vi "replaceTokens.vi"(8 "error in (no error)":errorcluster, 10 "Querry In":string, 11 "Goal in":refnum<class "Goal.lvclass">) -> (0 "error out":errorcluster, 2 "Query Out":string, 3 "Goal out":refnum<class "Goal.lvclass">)   [LabVIEW 2018, in "Goal.lvclass"]
uses:
  Goal.lvclass
  C:/GitRepos/Filthy-Lucre-Budgetizer/source/support/classes/UserEditableAmount/UserEditableAmount.lvclass
  Goal.lvclass/Goal.ctl
  WhichMonth/WhichMonth.lvclass
  Category/Category.lvclass
  UserEditableAmount/UserEditableAmount.lvclass
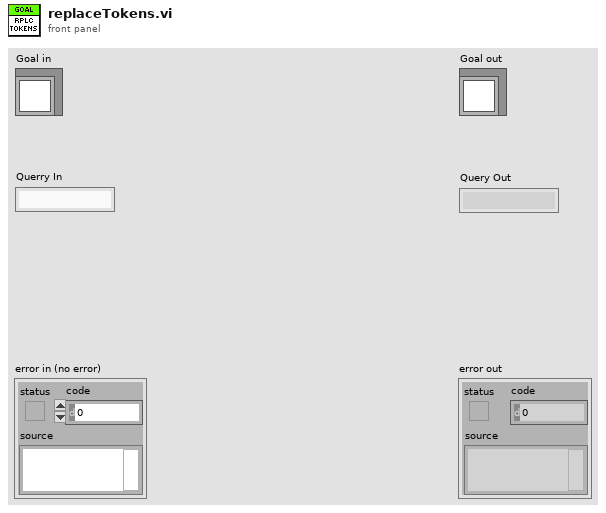
[diagram p1: front panel]
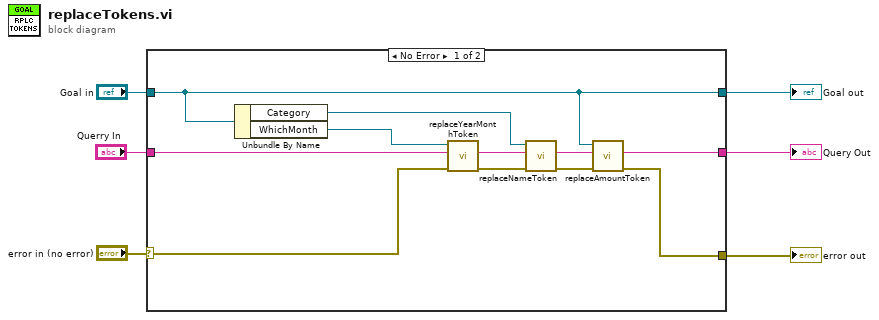
[diagram p0: block diagram]
diagram:
  n1 = case shown="No Error" "error in (no error)" {
    selector: "error in (no error)" -> [w16 w19]
    tunnel: [w9 w19] -> w5
    tunnel: [w7 w18] -> w3
    tunnel: "Goal in" -> [w7 w18]
    tunnel: [w8 _] -> w2
    tunnel: "Querry In" -> [w17 _]
    frame No Error {
      n2 = Unbundle By Name(w7) -> ("Category"=w14:refnum<class "Category.lvclass">, "WhichMonth"=w15:refnum<class "WhichMonth.lvclass">)
      n3 = call "replaceYearMonthToken.vi"("error in (no error)"=w16, "Query In"=w17, "WhichMonth in"=w15) -> ("error out"=w12:errorcluster, "Query Out"=w13:string)  [unwired: 6 in, 1 out]
      n4 = call "replaceNameToken.vi"("error in (no error)"=w12, "Query In"=w13, "Category in"=w14) -> ("error out"=w11:errorcluster, "Query Out"=w10:string)  [unwired: 6 in, 1 out]
      n5 = call "replaceAmountToken.vi"("error in (no error)"=w11, "Query In"=w10, "UserEditableAmount in"=w7) -> ("error out"=w9:errorcluster, "Query Out"=w8:string)  [unwired: 6 in, 1 out]
    }
    frame Error {
    }
  }
  "error out" <- w5
  "Goal out" <- w3
  "Query Out" <- w2
